vi "Lidar Encoder Counter.vi"   [LabVIEW 2010]
uses:
  Motor Encoder Global.vi
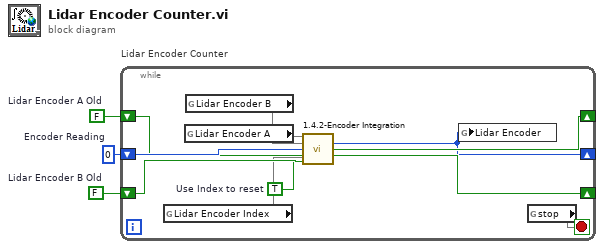
[diagram p0: block diagram]
diagram:
  w3 = 0  # Encoder Reading
  w2 = FALSE  # Lidar Encoder A Old
  w1 = FALSE  # Lidar Encoder B Old
  n1 = while "Lidar Encoder Counter" {
    shift-right: [w13] -> _
    shift-left: w2 -> [w12]
    shift-right: [w11] -> _
    shift-left: w1 -> [w10]
    shift-right: [w5] -> _
    shift-left: w3 -> [w14]
    stop <- w9 stop-if-true
    w4 = TRUE  # Use Index to reset
    n2 = global read "Motor Encoder Global.vi" "Lidar Encoder Index"() -> (w6)
    n3 = global read "Motor Encoder Global.vi" "Lidar Encoder A"() -> (w7)
    n4 = global read "Motor Encoder Global.vi" "Lidar Encoder B"() -> (w8)
    n5 = call "1.4.2-Encoder Integration.vi"("Encoder B"=w8, "Encoder A"=w7, 7:w14, "Encoder A Old"=w12, "Encoder B Old"=w10, 12:w4, "Encoder Index"=w6) -> ("Count Zeroed at Index"=w5:i32, "Encoder A Old (sReg)"=w13:bool, "Encoder B Old (sReg)"=w11:bool)  [unwired: 3 in, 3 out]
    n6 = global write "Motor Encoder Global.vi" "Lidar Encoder"(w5) -> ()
    n7 = global read "Motor Encoder Global.vi" "stop"() -> (w9)
  }
